vi "Page_Info_Write.vi"(6 "ctlReferences":T1, 8 "error in (no error)":errorcluster, 10 "Target filename":string, 11 "AB_Build in":refnum<class "AB_Build.lvclass">) -> (0 "error out":errorcluster, 3 "AB_Build out":refnum<class "AB_Build.lvclass">)   [LabVIEW 2020, in "AB_Build.lvclass"]
uses:
  <vilib>/AppBuilder/AB_Classes/Build/AB_Build.lvclass
  <resource>/Framework/Providers/Builds/AppBuilder/AB_UI_Page_Info_References.ctl
  <vilib>/AppBuilder/AB_Classes/Build/AB_Build.lvclass/AB_Build.ctl
  <vilib>/AppBuilder/AB_Classes/Destination/AB_Destination.lvclass
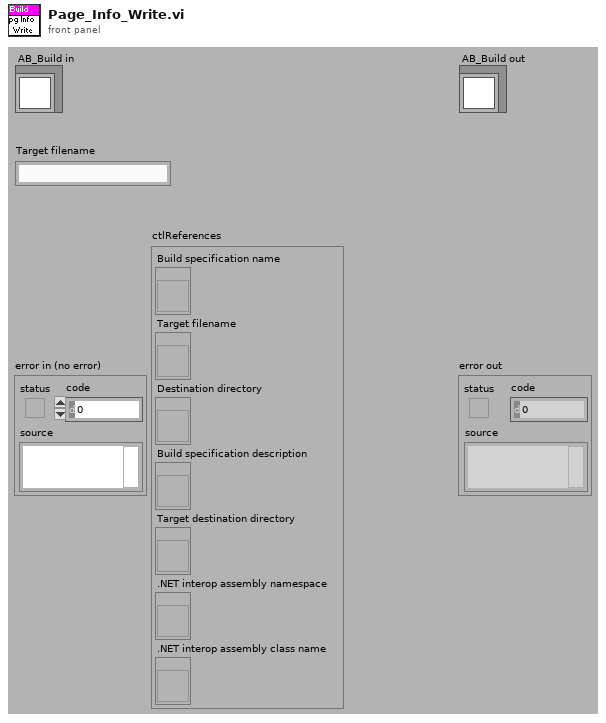
[diagram p1: front panel]
types:
  T1 = typedef "AB_UI_Page_Info_References.ctl" = cluster{"Build specification name":refnum<vi>, "Target filename":refnum<vi>, "Destination directory":refnum<vi>, "Build specification description":refnum<vi>, "Target destination directory":refnum<vi>, ".NET interop assembly namespace":refnum<vi>, ".NET interop assembly class name":refnum<vi>}
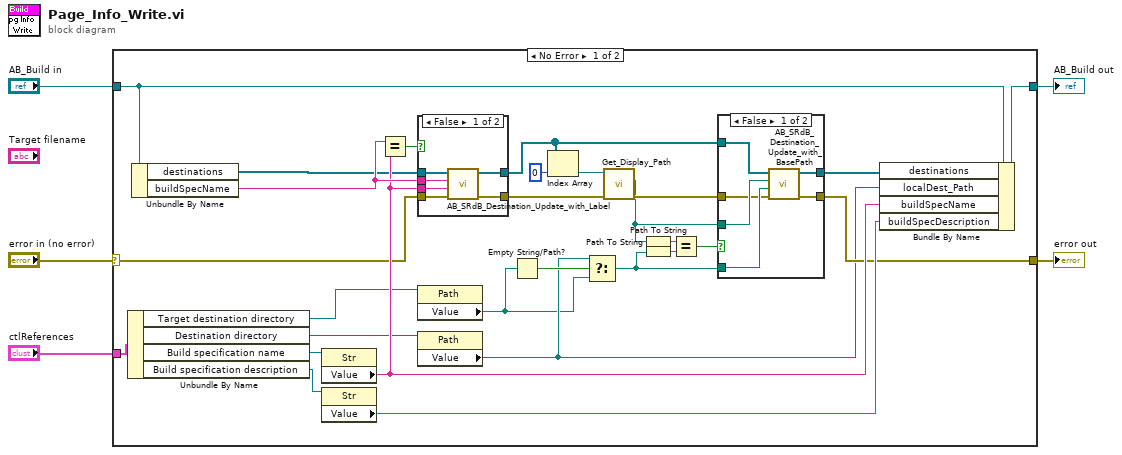
[diagram p0: block diagram]
diagram:
  n1 = case shown="No Error" "error in (no error)" {
    selector: "error in (no error)" -> [w14 w51]
    tunnel: [w13 w51] -> w4
    tunnel: [w30 w50] -> w2
    tunnel: "AB_Build in" -> [w28 w50]
    tunnel: "ctlReferences" -> [w33 _]
    frame No Error {
      n2 = Unbundle By Name(w33) -> ("Target destination directory"=w12:refnum<vi>, "Destination directory"=w18:refnum<vi>, "Build specification name"=w32:refnum<vi>, "Build specification description"=w31:refnum<vi>)
      n3 = Unbundle By Name(w28) -> ("destinations"=w24:refnum<class "AB_Destination.lvclass">[], "buildSpecName"=w26:string)
      n4 = property class="Str"(reference=w32) -> ("Value"=w25:string)  [unwired: 1 in, 2 out]
      n5 = property class="Str"(reference=w31) -> ("Value"=w29:string)  [unwired: 1 in, 2 out]
      n6 = Equal?(x=w26, y=w25) -> (x = y?=w27:bool)
      n7 = case shown="False" w27 {
        tunnel: w25 -> [w43 _]
        tunnel: w26 -> [w47 _]
        tunnel: w24 -> [w46 w49]
        tunnel: [w45 w48] -> w17
        tunnel: [w44 w49] -> w16
        tunnel: w14 -> [w42 w48]
        frame False {
          n8 = call <resource>:"AB_SRdB_Destination_Update_with_Label.vi"("error in (no error)"=w42, "new label"=w43, "old label"=w47, "ALL data in"=w46) -> ("error out"=w45:errorcluster, "ALL data out"=w44:refnum<class "AB_Destination.lvclass">[])  [unwired: 6 in]
        }
        frame True {
        }
      }
      n9 = property class="Path"(reference=w12) -> ("Value"=w9:path)  [unwired: 1 in, 2 out]
      n10 = property class="Path"(reference=w18) -> ("Value"=w10:path)  [unwired: 1 in, 2 out]
      n11 = Empty String/Path?(string/path=w9) -> (empty?=w11:bool)
      n12 = Index Array(array=w16, index=0) -> (element=w22:refnum<class "AB_Destination.lvclass">)
      n13 = Select(t=w10, s=w11, f=w9) -> (s? t:f=w8:path)
      n14 = call-dynamic "Get_Display_Path.vi"("error in (no error)"=w17, "AB_Destination in"=w22) -> ("error out"=w21:errorcluster, "displayPath"=w20:path)  [unwired: 7 in, 1 out]
      n15 = Path To String(path=w20) -> (string=w7:string)
      n16 = Path To String(path=w8) -> (string=w6:string)
      n17 = Equal?(x=w7, y=w6) -> (x = y?=w19:bool)
      n18 = case shown="False" w19 {
        tunnel: w21 -> [w34 w40]
        tunnel: w8 -> [w38 _]
        tunnel: w20 -> [w39 _]
        tunnel: w16 -> [w35 w41]
        tunnel: [w37 w41] -> w15
        tunnel: [w36 w40] -> w13
        frame False {
          n19 = call <resource>:"AB_SRdB_Destination_Update_with_BasePath.vi"("error in (no error)"=w34, "new base path"=w38, "old base path"=w39, "ALL data in"=w35) -> ("error out"=w36:errorcluster, "ALL data out"=w37:refnum<class "AB_Destination.lvclass">[])  [unwired: 6 in]
        }
        frame True {
        }
      }
      n20 = Bundle By Name(cluster=w28, "destinations"=w15, "localDest_Path"=w10, "buildSpecName"=w25, "buildSpecDescription"=w29) -> (w30:refnum<class "AB_Build.lvclass">)
    }
    frame Error {
    }
  }
  "error out" <- w4
  "AB_Build out" <- w2
